vi "Start Call (Exe-Args).vi"(6 "Event References":T1, 7 "Configuration":refnum<class "configuration.lvclass">, 8 "error in":errorcluster, 9 "Working Directory (default <Not A Path> - System Default)":path=path "" caption="Working Directory", 10 "Arguments (Default: Empty)":string[](array[string]), 11 "Executable Path":path) -> (0 "error out":errorcluster, 3 "New ASE Handle":refnum<class "ase.lvclass">)   [LabVIEW 2020, in "serenial.io-ase.lvlib" / "ase.lvclass"]
doc: "<B>Start an Asynchronous System Executable Call</B>\n\nThe absolute path to the executable should be supplied.\n\nThe User Events References to generate the \"Did Launch\", \"Standard Output\", \"Standard Error\" and \"Did Exit\" events can be supplied or omitted as required. <B>Ensure that the event registration process for any User Events passed to this VI has already been undertaken</B>.\n\nArguments that are to be passed to the executable are specified in an array. Ensure that each argument specifier or value is in a different array element. E.g. to call the ping executable with the arguments \"-n 10 localhost\" use the element values [ -n, 10, localhost]. See the \"examples of the exe-args style calls\" from the boost documentation at https://www.boost.org/doc/libs/1_77_0/doc/html/boost_process/design.html#boost_process.design.arg_cmd_style.\n\n\nThe configuration class allows for override of certain behaviours such as the regular expression used to match the breaks in the Standard Out and Standard Error to be specified.\n\nThis VI generates the following errors:\n-4601: Poorly formatted/incorrect Regular Expression supplied.\n-5691000: Internal Library Error. <Check Error Message for more details>\n-5691301: Unable to launch the executable. <Check Error Message for more details>\n-5691305: Executable paths parameter cannot be an empty value."
uses:
  ase.lvclass
  Event References.ctl
  Standard Output.ctl
  Standard Error.ctl
  Did Exit.ctl
  configuration/configuration.lvclass
  ase.lvclass/ase.ctl
  Error Empty Executable Name.vi
  Check Shared Library Version.vi
  Merge Call Library Errors.vi
  Trim Whitespace.vi
  Error Internal Library Implementation Error.vi
  <vilib>/Utility/error.llb/Error Cluster From Error Code.vi
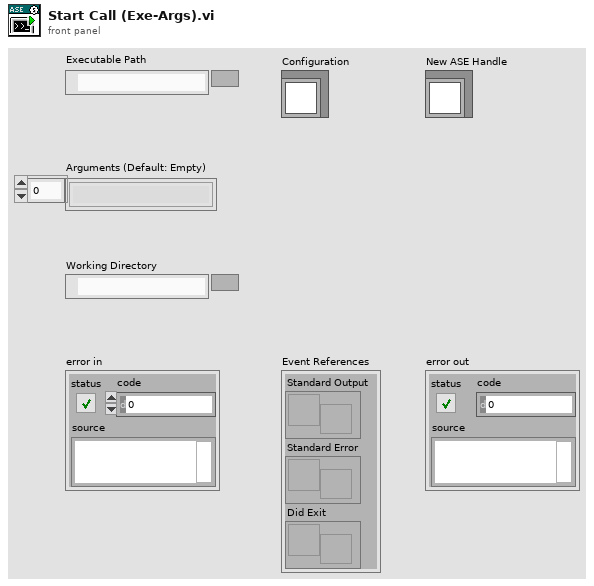
[diagram p1: front panel]
types:
  T1 = typedef "serenial.io-ase.lvlib/ase.lvclass/Event References.ctl" = cluster{"Standard Output":refnum<user-event>, "Standard Error":refnum<user-event>, "Did Exit":refnum<user-event>}
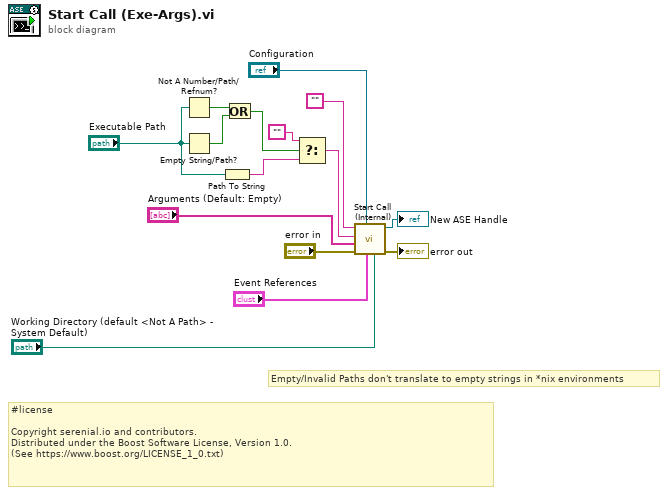
[diagram p0: block diagram]
diagram:
  # "#license\n\nCopyright serenial.io and contributors.\nDistributed under the Boost Software License, Version 1.0.\n(See https://www.boost.org/LICENSE_1_0.txt)"
  # "Empty/Invalid Paths don't translate to empty strings in *nix environments"
  n1 = Not A Number/Path/Refnum?(number/path/refnum="Executable Path") -> (NaN/Path/Refnum?=w9:bool)
  n2 = Empty String/Path?(string/path="Executable Path") -> (empty?=w10:bool)
  n3 = Path To String(path="Executable Path") -> (string=w4:string)
  n4 = Or(x=w9, y=w10) -> (x .or. y?=w7:bool)
  n5 = Select(t="" ("Empty String Constant"), s=w7, f=w4) -> (s? t:f=w3:string)
  n6 = call "Start Call (Internal).vi"("Working Directory (default <Not A Path> - System Default)"="Working Directory (default <Not A Path> - System Default)", "Event References"="Event References", "Configuration"="Configuration", "error in"="error in", "Arguments"="Arguments (Default: Empty)", "Exe"=w3, "Command"="" ("Empty String Constant")) -> ("error out"=→"error out":errorcluster, "New ASE Handle"=→"New ASE Handle":refnum<class "ase.lvclass">)  [unwired: 3 in]
